vi "PH_PSDBController.set Shot ID.vi"(0 "i ref in":refnum<vi>, 5 "error in":errorcluster) -> (14 "i ref out":refnum<vi>, 19 "error out":errorcluster)   [LabVIEW 2014, in "PH_PSDBController.lvlib"]
doc: "This VI gets the current Shot ID and provides this information."
uses:
  PH_PSDBController.lvlib
  PH_Basics/PH_PSDBWriter/PH_PSDBWriter.Data Status.ctl
  CSlibraries-extern/psdb_lv/PSDB.lvlib
  PH_Basics/PH_PSDBWriter/PH_PSDBWriter.lvlib
  CSlibraries-extern/DimLVEvent/LVDimInterface/LVDimInterface.lvlib
  PH_Basics/PH_Common/PH_Common.lvlib
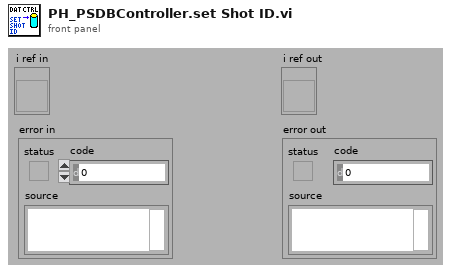
[diagram p1: front panel]
types:
  T1 = typedef "PH_PSDBController.lvlib/PH_PSDBController.i attribute.ctl" = cluster{"GUI Refs":cluster{"Data Status":refnum<vi>, "Current Shot ID":refnum<vi>, "active Subsystems":refnum<vi>, "Experiment Description":refnum<vi>, "Shot Comment":refnum<vi>, "Experiment":refnum<vi>, "Shottype":refnum<vi>, "Sequencer SM State":refnum<vi>, "Instances with Errors":refnum<vi>}, "Service ID Shot ID":i32, "Service ID wanted Subsystem":i32, "Data Status":T2, "Shotinformation":cluster{"Current Experiment ID":i32, "Current Shot Type":i32, "Current Comment":string}, "Data taking?":bool, "Service ID current Shottype":i32, "Service ID current Experiment":i32, "Service ID currentShot Comment":i32, "Service ID possible Shottypes":i32, "Service ID possible Experiments":i32, "possible Experiments":T3[], "possible Shottypes":T3[], "List":cluster{"Info":cluster{"Instance":string, "Data Status":T2}[], "GUI Ref":refnum<vi>, "Classname":string}[], "Subsystems Off?":cluster{"PHELIX_Beamline_fs_YLF_BL_Status":bool, "PHELIX_Beamline_ns_BL_Status":bool, "PHELIX_Beamline_PA_Input_BL_Status":bool, "PHELIX_Beamline_PA_MA_BL_Status":bool, "PHELIX_Beamline_MA_Z6_BL_Status":bool, "PHELIX_Beamline_MA_LB_BL_Status":bool, "PHELIX_Beamline_PA_LL_BL_Status":bool}, "PSDB Credentials":T4}
  T2 = typedef "PH_PSDBWriter.lvlib/PH_PSDBWriter.Data Status.ctl" = i16
  T3 = typedef "PSDB.lvlib/PSDB_Info.ctl" = cluster{"Name":string, "Description":string, "ID":i32}
  T4 = typedef "PH_Common.lvlib/PH_Connection.PSDB Credentials.ctl" = cluster{"PW":string, "ID":string, "DS":string}
  T5 = typedef "NI_Database_API.lvlib/Conn ObjectReference.ctl" = refnum<k1>
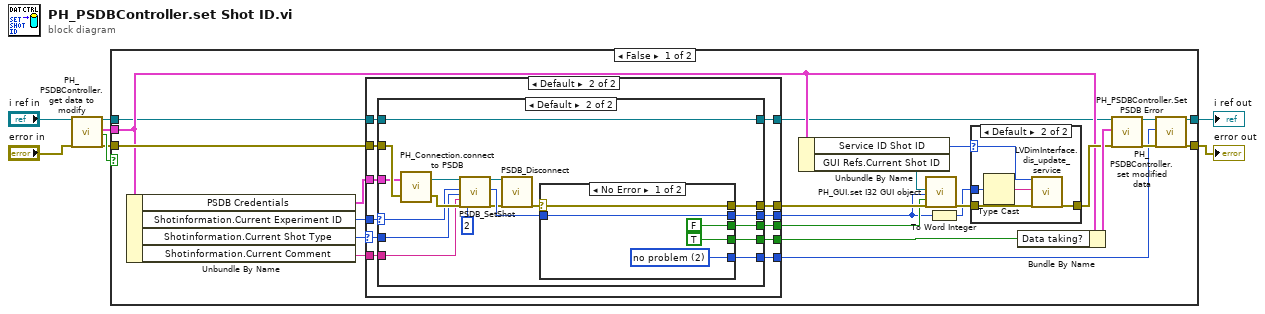
[diagram p0: block diagram]
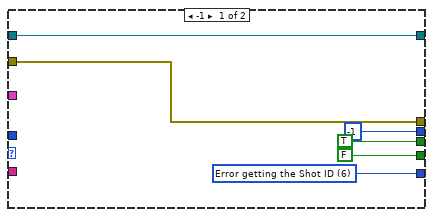
[diagram p2: hidden frame]
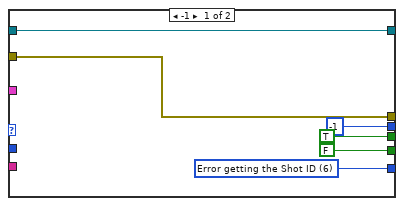
[diagram p3: hidden frame]
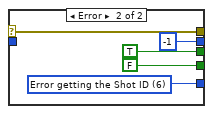
[diagram p4: hidden frame]
diagram:
  n1 = call "PH_PSDBController.get data to modify.vi"("i ref in"="i ref in", "error in (no error)"="error in") -> ("i ref out"=w3:refnum<vi>, "i attribute"=w1:T1, "timed out"=w4:bool, "error out"=w2:errorcluster)  [unwired: 14 in]
  n2 = case shown="False" w4 {
    tunnel: w1 -> [w12 _]
    tunnel: w2 -> [w24 w90]
    tunnel: [w18 w90] -> w7
    tunnel: w3 -> [w11 w91]
    tunnel: [w20 w91] -> w8
    frame False {
      n3 = Unbundle By Name(w12) -> ("PSDB Credentials"=w9:T4, "Shotinformation.Current Experiment ID"=w23:i32, "Shotinformation.Current Shot Type"=w22:i32, "Shotinformation.Current Comment"=w30:string)
      n4 = case shown="Default" w22 {
        selector: w22 -> [_ w41]
        tunnel: [w35 w49] -> w17
        tunnel: w30 -> [_ w48]
        tunnel: [FALSE w47] -> w29
        tunnel: [w33 w46] -> w26
        tunnel: [-1 ("shot_id") w45] -> w15
        tunnel: [TRUE w44] -> w25
        tunnel: w24 -> [w33 w43]
        tunnel: w23 -> [_ w42]
        tunnel: w11 -> [w32 w40]
        tunnel: [w32 w39] -> w10
        tunnel: w9 -> [_ w38]
        frame -1 {
          w35 = T2 6 items=["no info", "no Data collection", "no problem", "Error getting the instance ID", "Error writing Data to data base", "Error concerning the subsystem", "Error getting the Shot ID"] ("Data Status")
        }
        frame Default {
          n5 = case shown="Default" w42 {
            selector: w42 -> [_ w61]
            tunnel: [w52 w73] -> w49
            tunnel: w41 -> [_ w60]
            tunnel: w48 -> [_ w67]
            tunnel: [FALSE w66] -> w47
            tunnel: [w55 w64] -> w46
            tunnel: [-1 ("shot_id") w63] -> w45
            tunnel: [TRUE w62] -> w44
            tunnel: w43 -> [w55 w58]
            tunnel: w40 -> [w50 w59]
            tunnel: [w50 w59] -> w39
            tunnel: w38 -> [_ w57]
            frame -1 {
              w52 = T2 6 items=["no info", "no Data collection", "no problem", "Error getting the instance ID", "Error writing Data to data base", "Error concerning the subsystem", "Error getting the Shot ID"] ("Data Status")
            }
            frame Default {
              n6 = call "PH_Connection.connect to PSDB.vi"("error in"=w58, "PSDB Credentials"=w57) -> ("error out"=w69:errorcluster, "connection reference"=w68:T5)
              n7 = call "PSDB_SetShot.vi"("connection reference"=w68, "experiment_id"=w61, "shottype_id"=w60, "description"=w67, "error in (no error)"=w69, "sysversion (1)"=u32 2) -> ("connection reference out"=w70:T5, "shot_id"=w72:i32, "error out"=w71:errorcluster)  [unwired: 11 in]
              n8 = call "PSDB_Disconnect.vi"("connection reference"=w70, "error in (no error)"=w71) -> ("error out"=w65:errorcluster)  [unwired: 17 in]
              n9 = case shown="No Error" w65 {
                selector: w65 -> [w75 w80]
                tunnel: [w78 w83] -> w73
                tunnel: w72 -> [w76 _]
                tunnel: [TRUE FALSE] -> w66
                tunnel: [w76 -1 ("shot_id")] -> w63
                tunnel: [w75 w80] -> w64
                tunnel: [FALSE TRUE] -> w62
                frame No Error {
                  w78 = T2 2 items=["no info", "no Data collection", "no problem", "Error getting the instance ID", "Error writing Data to data base", "Error concerning the subsystem"] ("Data Status")
                }
                frame Error {
                  w83 = T2 6 items=["no info", "no Data collection", "no problem", "Error getting the instance ID", "Error writing Data to data base", "Error concerning the subsystem", "Error getting the Shot ID"] ("Data Status")
                }
              }
            }
          }
        }
      }
      n10 = Unbundle By Name(w12) -> ("Service ID Shot ID"=w14:i32, "GUI Refs.Current Shot ID"=w13:refnum<vi>)
      n11 = call "PH_GUI.set I32 GUI object.vi"("I32 GUI Ref"=w13, "value"=w15, "blinking (false)"=w25, "error in (no error)"=w26) -> ("error out"=w28:errorcluster)  [unwired: 15 in]
      n12 = To Word Integer(number=w15) -> (16bit integer=w16:i16)
      n13 = case shown="Default" w14 {
        selector: w14 -> [_ w87]
        tunnel: [w84 w88] -> w27
        tunnel: w28 -> [w84 w89]
        tunnel: w16 -> [_ w85]
        frame -1 {
        }
        frame Default {
          n14 = Type Cast(x=w85) -> (*(type *) &x=w86:string)  [unwired: 1 in]
          n15 = call "LVDimInterface.dis_update_service.vi"("my_serviceID"=w87, "data"=w86, "error in (no error)"=w89) -> ("error out"=w88:errorcluster)  [unwired: 14 in, 2 out]
        }
      }
      n16 = Bundle By Name(cluster=w12, "Data taking?"=w29) -> (w31:T1)
      n17 = call "PH_PSDBController.set modified data.vi"("i ref in"=w10, "i attribute"=w31, "error in (no error)"=w27) -> ("i ref out"=w21:refnum<vi>, "error out"=w19:errorcluster)  [unwired: 15 in]
      n18 = call "PH_PSDBController.Set PSDB Error.vi"("i ref in"=w21, "Data Status"=w17, "error in"=w19) -> ("i ref out"=w20:refnum<vi>, "error out"=w18:errorcluster)  [unwired: 15 in]
    }
    frame True {
    }
  }
  "i ref out" <- w8
  "error out" <- w7
